vi "to string 3.3.vi"(8 "error in":errorcluster, 10 "data in":string, 11 "Shared Memory configuration in":refnum<class "Shared Memory configuration.lvclass">) -> (0 "error out":errorcluster, 2 "data out":string, 3 "Shared Memory configuration out":refnum<class "Shared Memory configuration.lvclass">)   [LabVIEW 2013, in "Shared Memory configuration.lvclass"]
uses:
  Shared Memory configuration.lvclass
  Shared Memory configuration.lvclass/Shared Memory configuration.ctl
  <vilib>/NI/Configuration Framework/serializable configuration/NISE_CEF_serializable configuration.lvclass
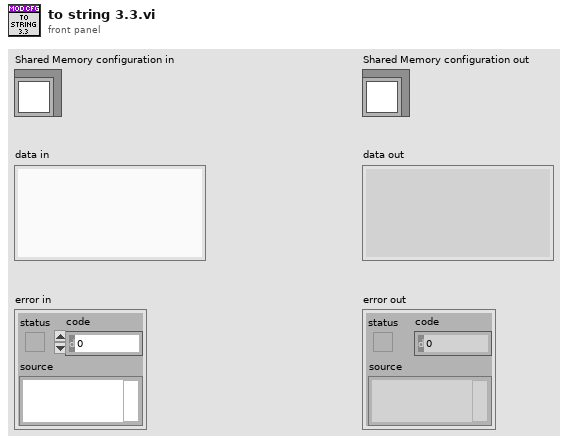
[diagram p1: front panel]
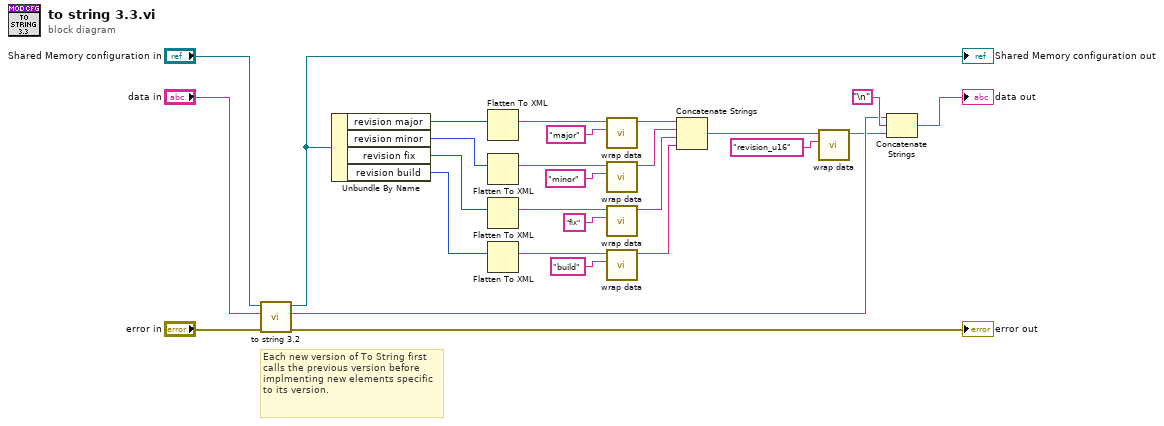
[diagram p0: block diagram]
diagram:
  # "Each new version of To String first calls the previous version before implmenting new elements specific to its version."
  n1 = call "to string 3.2.vi"("error in"="error in", "data in"="data in", "Shared Memory configuration in"="Shared Memory configuration in") -> ("error out"=→"error out":errorcluster, "data out"=w21:string, "Shared Memory configuration out"=w5:refnum<class "Shared Memory configuration.lvclass">)  [unwired: 6 in]
  "Shared Memory configuration out" <- w5
  n2 = Unbundle By Name(w5) -> ("revision major"=w4:u16, "revision minor"=w3:u16, "revision fix"=w2:u16, "revision build"=w1:u16)
  n3 = Flatten To XML(anything=w4) -> (xml string=w16:string)
  n4 = Flatten To XML(anything=w3) -> (xml string=w13:string)
  n5 = Flatten To XML(anything=w2) -> (xml string=w14:string)
  n6 = Flatten To XML(anything=w1) -> (xml string=w15:string)
  n7 = call <vilib>:"wrap data.vi"("identifier"="major", "data to wrap"=w16) -> ("wrapped data"=w11:string)  [unwired: 9 in]
  n8 = call <vilib>:"wrap data.vi"("identifier"="minor", "data to wrap"=w13) -> ("wrapped data"=w7:string)  [unwired: 9 in]
  n9 = call <vilib>:"wrap data.vi"("identifier"="fix", "data to wrap"=w14) -> ("wrapped data"=w10:string)  [unwired: 9 in]
  n10 = call <vilib>:"wrap data.vi"("identifier"="build", "data to wrap"=w15) -> ("wrapped data"=w9:string)  [unwired: 9 in]
  n11 = Concatenate Strings(w11, w7, w10, w9) -> (w8:string)
  n12 = call <vilib>:"wrap data.vi"("identifier"="revision_u16", "data to wrap"=w8) -> ("wrapped data"=w6:string)  [unwired: 9 in]
  n13 = Concatenate Strings(w21, "\n", w6) -> (→"data out":string)
